vi "Set Pure Pursuit Path.vi"(8 "error in (no error)":errorcluster, 10 "Reverse? (F)":bool, 11 "Path":cluster{dbl, "interpolation value":dbl}[](array[cluster])) -> (0 "error out":errorcluster)   [LabVIEW 2017]
doc: "This VI notifies the subsystem to the new setpoint."
uses:
  Pure Pursuit/Pure Pursuit.lvlib
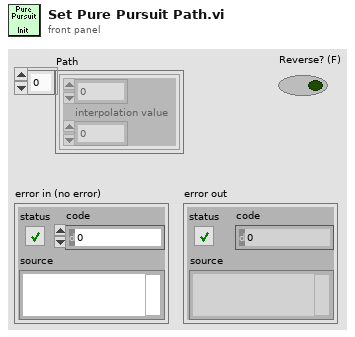
[diagram p1: front panel]
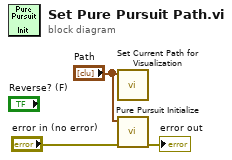
[diagram p0: block diagram]
diagram:
  n1 = call "Set Current Path for Visualization.vi"("Path"="Path") -> ()  [unwired: 11 in]
  n2 = call "Pure Pursuit Initialize.vi"("error in (no error)"="error in (no error)", "Path"="Path") -> ("error out"=→"error out":errorcluster)  [unwired: 9 in]
